vi "Read database.vi"(0 "table":string="CODMn", 1 "显示项":string[](array[string]), 5 "测量模式":T1(ring), 11 "error in (no error)":errorcluster caption="错误输入（无错误）") -> (4 "表格":string[][](table), 8 "foretime":string, 10 "lasttime":string, 15 "error out":errorcluster caption="错误输出")   [LabVIEW 2016, in "斯坦道总磷总氮.lvlib"]
uses:
  <vilib>/Utility/sysdir.llb/System Directory Type.ctl
  <vilib>/addons/database/Connection.llb/DB Tools Open Connec (String).vi
  <vilib>/addons/database/_DB Variant To Data/Database Variant To Data.xnode
  <vilib>/addons/database/NI_Database_API.lvlib
panel:
  out "电子表格字符串":string
  out "SQL":string="where 时间 between #2020/03/27 14:26:18 # and #2020/04/26 14:26:18# order by 时间 desc"
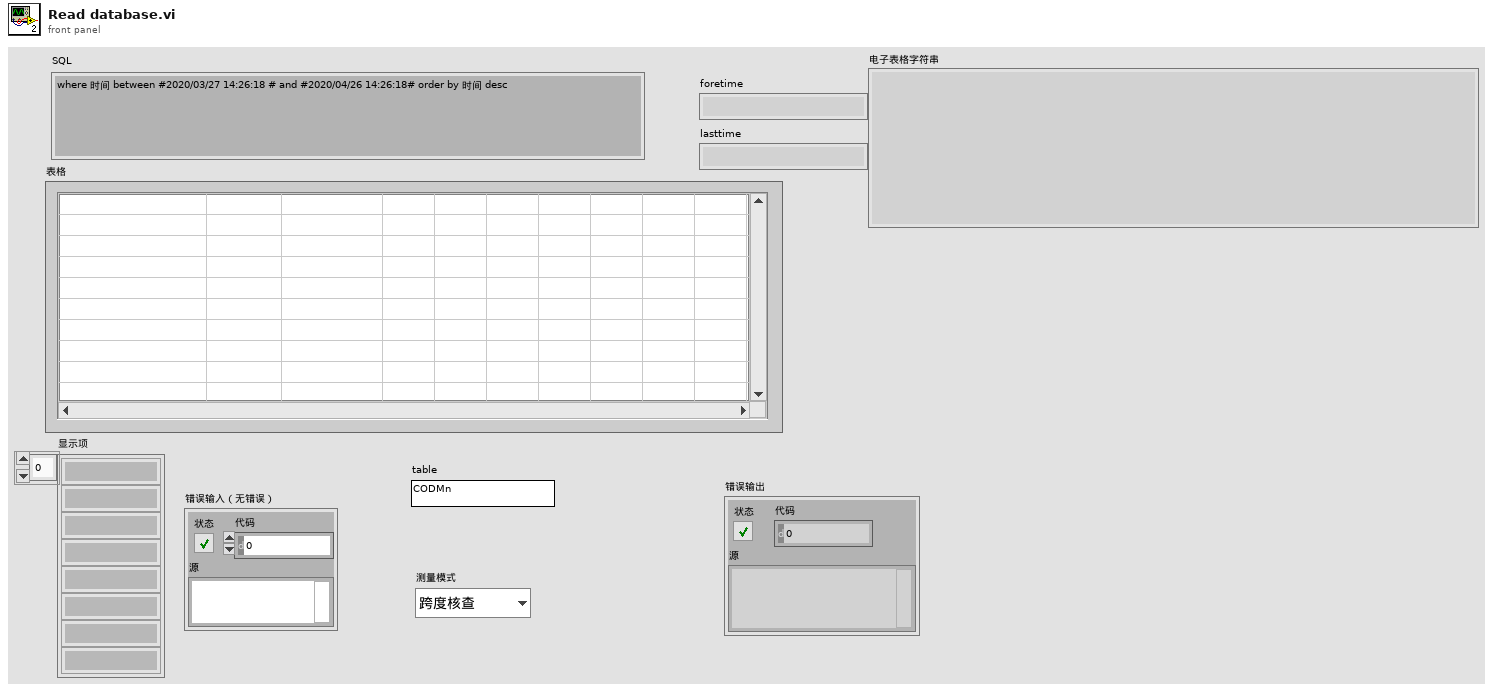
[diagram p1: front panel]
types:
  T1 = enum16{"跨度核查", "水样测量", "零点核查", "标样核查", "加标回收", "快捷测试", "空白校准", "标样校准"}
  T2 = typedef "System Directory Type.ctl" = i32
  T3 = typedef "NI_Database_API.lvlib/Conn ObjectReference.ctl" = refnum<k1>
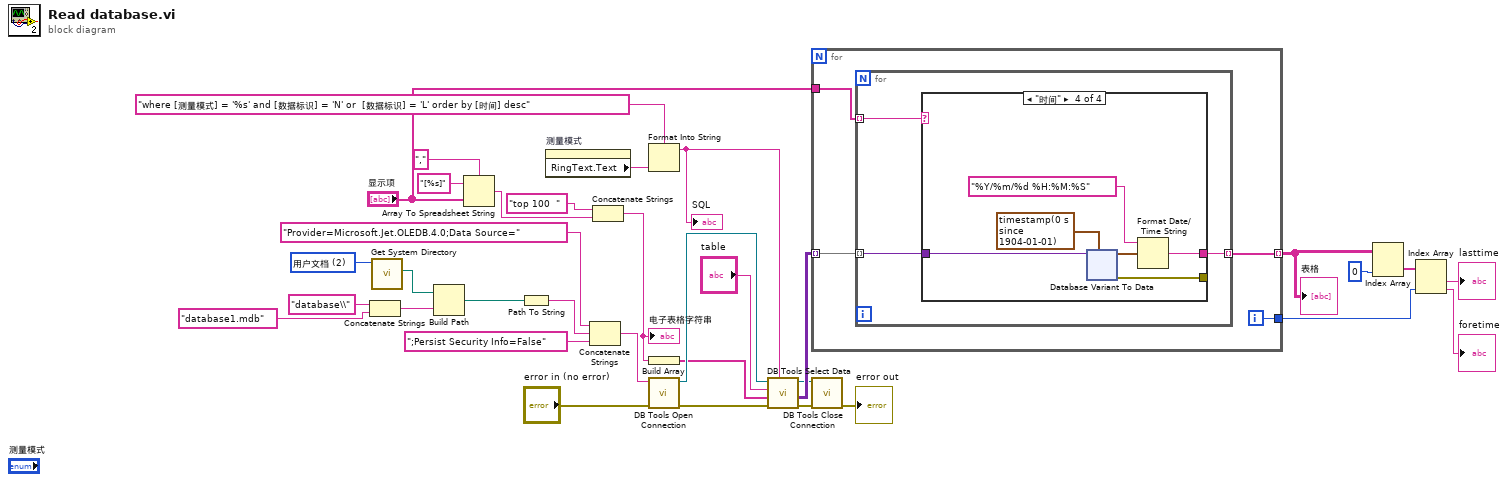
[diagram p0: block diagram]
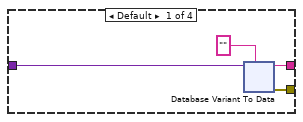
[diagram p2: hidden frame]
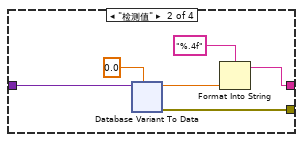
[diagram p3: hidden frame]
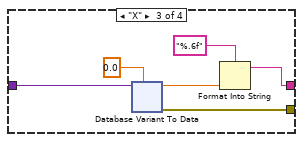
[diagram p4: hidden frame]
diagram:
  w24 = T2 2 items=["用户目录"=0, "用户桌面"=1, "用户文档"=2, "用户应用程序数据"=3, "用户设置"=4, "用户临时目录"=5, "公共文档"=6, "公共应用程序数据"=7, "公共设置"=8, "公共缓存"=13, "系统核心库"=9, "系统安装库"=10, "应用程序文件"=11, "启动盘根目录"=12] ("system directory type")
  n1 = Concatenate Strings("database\\" ("名称或相对路径"), "database1.mdb" ("database")) -> (w20:string)
  n2 = call <vilib>:"Get System Directory.vi"("system directory type"=w24) -> ("system directory"=w23:path)  [unwired: 10 in]
  n3 = Build Path(base path=w23, name or relative path=w20) -> (appended path=w25:path)
  n4 = Array To Spreadsheet String(delimiter (Tab)="," ("分隔符(Tab)"), array="显示项", 3:"[%s]" ("格式字符串")) -> (spreadsheet string=w6:string)
  n5 = Path To String(path=w25) -> (string=w26:string)
  n6 = property on="测量模式" class="Enum (严格)"() -> ("RingText.Text"=w1:string)  [unwired: 2 in, 2 out]
  n7 = Concatenate Strings("Provider=Microsoft.Jet.OLEDB.4.0;Data Source=", w26, ";Persist Security Info=False") -> (w22:string)
  n8 = Concatenate Strings("top 100  " ("字符串"), w6) -> (w4:string)
  "电子表格字符串" <- w4
  n9 = Format Into String(format string="where [测量模式] = '%s' and [数据标识] = 'N' or  [数据标识] = 'L' order by [时间] desc" ("格式字符串"), w1) -> (resulting string=w9:string)  [unwired: 2 in, 1 out]
  "SQL" <- w9
  n10 = Build Array(w4) -> (w5:string[])
  n11 = call-poly <vilib>:"DB Tools Open Connection.vi"("error in (no error)"="error in (no error)", "connection information"=w22) -> ("error out"=w33:errorcluster, "connection reference"=w34:T3)  [unwired: 6 in]
  n12 = call <vilib>:"DB Tools Select Data.vi"("condition"=w9, "error in (no error)"=w33, "columns"=w5, "table"="table", "connection reference"=w34) -> ("error out"=w32:errorcluster, "data"=w18:variant[][], "connection reference out"=w17:T3)  [unwired: 1 in]
  n13 = for {
    tunnel: w18 -> [w38] mode=indexing
    tunnel: [w37] -> w15 mode=indexing
    tunnel: [w36] -> w11
    tunnel: "显示项" -> [w35]
    i -> [w36]
    n14 = for {
      tunnel: w38 -> [w40] mode=indexing
      tunnel: [w41] -> w37 mode=indexing
      tunnel: w35 -> [w39] mode=indexing
      n15 = case shown="\"时间\"" w39 {
        tunnel: w40 -> [w45 w83 w121 w159]
        tunnel: [w42 w79 w117 w155] -> w41
        tunnel: [w43 w82 w120 w154] -> _
        frame Default {
          n16 = xnode "Database Variant To Data"("database variant"=w45, "type"="") -> ("data"=w42:string, "error out"=w43:errorcluster)  [unwired: 1 in]
        }
        frame "检测值" {
          n17 = xnode "Database Variant To Data"("database variant"=w83, "type"=0.0) -> ("data"=w80:dbl, "error out"=w82:errorcluster)  [unwired: 1 in]
          n18 = Format Into String(format string="%.4f" ("格式字符串"), w80) -> (resulting string=w79:string)  [unwired: 2 in, 1 out]
        }
        frame "X" {
          n19 = xnode "Database Variant To Data"("database variant"=w121, "type"=0.0) -> ("data"=w118:dbl, "error out"=w120:errorcluster)  [unwired: 1 in]
          n20 = Format Into String(format string="%.6f" ("格式字符串"), w118) -> (resulting string=w117:string)  [unwired: 2 in, 1 out]
        }
        frame "时间" {
          n21 = xnode "Database Variant To Data"("database variant"=w159, "type"=timestamp(0 s since 1904-01-01) ("当前时间")) -> ("data"=w158:timestamp, "error out"=w154:errorcluster)  [unwired: 1 in]
          n22 = Format Date/Time String(time format string (%c)="%Y/%m/%d %H:%M:%S" ("时间格式字符串(%c)"), seconds (now)=w158) -> (date/time string=w155:string)  [unwired: 1 in]
        }
      }
    }
  }
  "表格" <- w15
  n23 = call <vilib>:"DB Tools Close Connection.vi"("error in (no error)"=w32, "connection reference"=w17) -> ("error out"=→"error out":errorcluster)  [unwired: 5 in]
  n24 = Index Array(array=w15, index (col)=0 ("禁用的索引 (列)")) -> (element=w14:string[])  [unwired: 1 in]
  n25 = Index Array(array=w14, index #2=w11) -> (element #1=→"lasttime":string, element #2=→"foretime":string)  [unwired: 1 in]
